vi "New Card Setup 2.vi"(0 "Yokogawa WT500 in":refnum<class "Yokogawa WT500.lvclass">, 5 "Card Array":bool[](array[boolean]), 11 "error in (no error)":errorcluster) -> (4 "Yokogawa WT500 out":refnum<class "Yokogawa WT500.lvclass">, 6 "decimal integer string":string[](array[string]), 8 "Continuous?":bool, 10 "Card chosen":i32, 14 "Time Cluster":T1, 15 "error out":errorcluster)   [LabVIEW 2012, in "Universal Power Meter.lvlib" / "Yokogawa WT500.lvlib" / "Yokogawa WT500.lvclass"]
uses:
  Yokogawa WT500.lvclass
  Universal Power Meter class/Universal Power Meter.lvclass
panel:
  in  "Current Sensor Ratio(mV/A) (10.0000)":dbl=10.0 min=0.0001 max=99999.9999 step=0.0001 format="%.4f"
  in  "Voltage Range (8: 1000V)":u16(ring)=8 items=["AUTO", "15", "30", "60", "100", "150", "300", "600", "1000", "7.5", "15", "30", "50", "75", "150", "300", "500"]
  in  "Current Range (7: 40A)":u16(ring)=7 items=["AUTO", "500 mA", "1 A", "2 A", "5 A", "10 A", "20 A", "40 A", "S-AUTO", "50 mV", "100 mV", "200 mV", "500 mV", "1 V", "2 V", "5 V", "10 V", "250 mA", "500 mA", "1 A", "2.5 A", "5 A", "10 A", "20 A", "25 mV", "50 mV", "100 mV", "250 mV", "500 mV", "1 V", "2.5 V", "5 V"]
  in  "Play Button":bool
  in  "Card to Start":u16(ring) items=["1", "2", "3"]
  in  "Measurement":enum32{"Continuous", "Timed"}(radio)
  in  "Measurement Time":dbl format="%<%H:%M:%S>t"
  in  "Warm Up Time":dbl format="%<%H:%M:%S>t"
  out "A Range (9: 5A) 2":u16(ring)=9 items=["AUTO", "10 mA", "20 mA", "50 mA", "100 mA", "200 mA", "500 mA", "1 A", "2 A", "5 A", "10 A", "20 A", "50 A", "S-AUTO", "50 mV", "100 mV", "250 mV", "500 mV", "1 V", "2.5 V", "5 V", "10 V"]
  out "V Range (12: 1000) 2":u16(ring)=9 items=["AUTO", "1.5", "3", "6", "10", "15", "30", "60", "100", "150", "300", "600", "1000"]
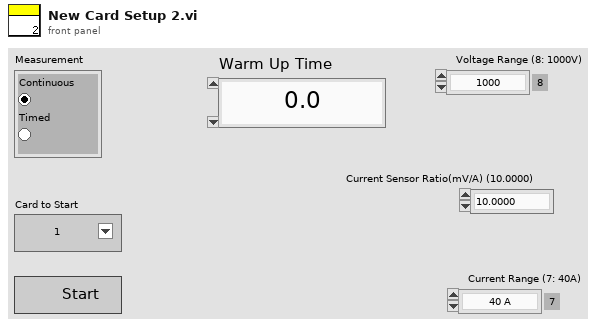
[diagram p1: front panel]
types:
  T1 = cluster{"Warm Up Time":dbl, "Measurement Time":dbl}
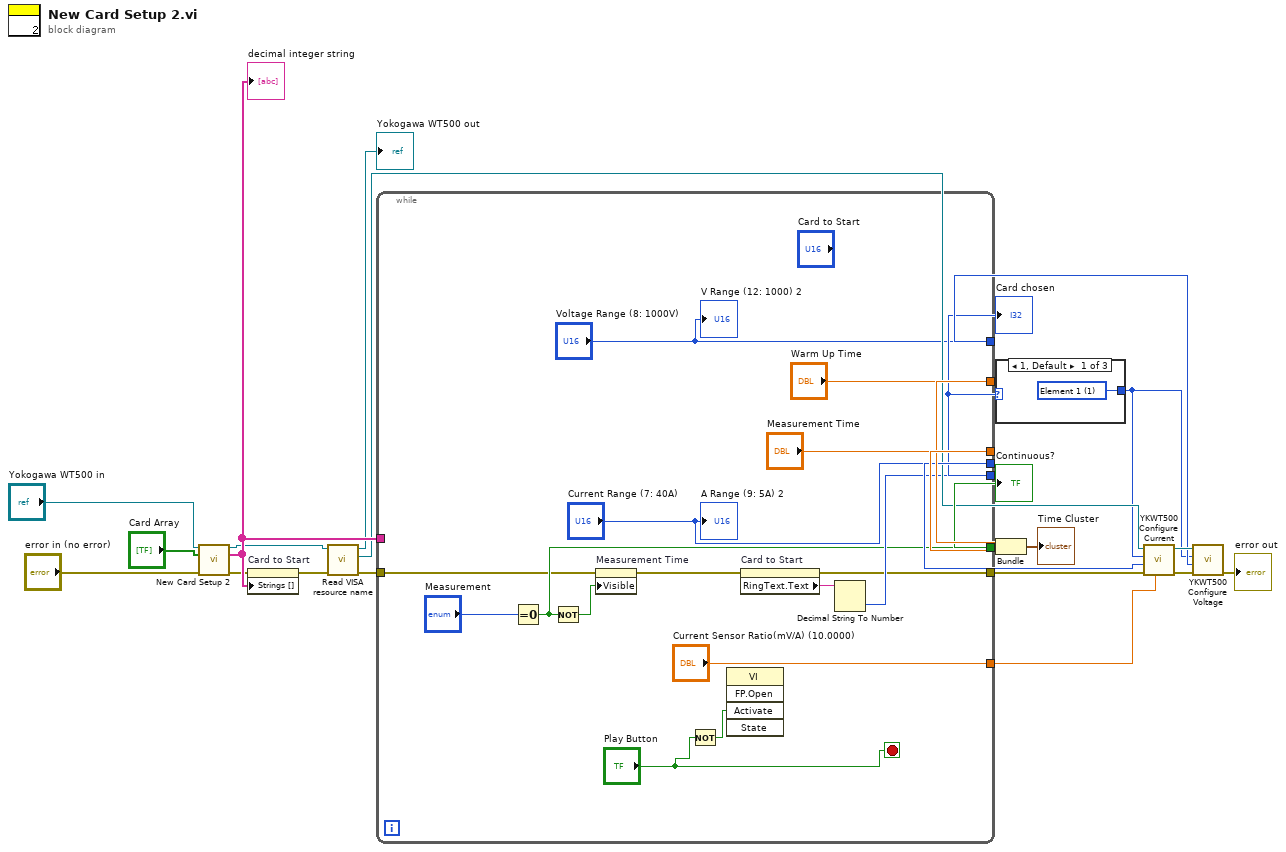
[diagram p0: block diagram]
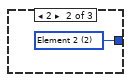
[diagram p2: hidden frame]
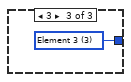
[diagram p3: hidden frame]
diagram:
  n1 = call-parent "New Card Setup 2.vi"("Generic Instrument in"="Yokogawa WT500 in", "Card Array"="Card Array", "error in (no error)"="error in (no error)") -> ("Generic Instrument out"=w9:refnum<class "Yokogawa WT500.lvclass">, "decimal integer string"=w18:string[], "error out"=w17:errorcluster)  [unwired: 7 in, 3 out]
  "decimal integer string" <- w18
  n2 = property on="Card to Start" class="Ring (strict)"(error in=w17, "Strings []"=w18) -> (error out=w7:errorcluster)  [unwired: 1 in, 1 out]
  n3 = call-dynamic "Read VISA resource name.vi"("error in (no error)"=w7, "Generic Instrument in"=w9) -> ("error out"=w6:errorcluster, "VISA resource name"=w5:refnum<visa-resource-name>, "Generic Instrument out"=→"Yokogawa WT500 out":refnum<class "Yokogawa WT500.lvclass">)  [unwired: 7 in]
  n4 = while {
    tunnel: [w37] -> w4
    tunnel: ["Measurement Time"] -> w20
    tunnel: ["Warm Up Time"] -> w19
    tunnel: [w33] -> w15
    tunnel: w18 -> [_]
    tunnel: w6 -> [w31]
    tunnel: [w29] -> w1
    tunnel: ["Current Range (7: 40A)"] -> w12
    tunnel: ["Voltage Range (8: 1000V)"] -> w11
    tunnel: ["Current Sensor Ratio(mV/A) (10.0000)"] -> w10
    stop <- "Play Button" stop-if-true
    n5 = Equal To 0?(x="Measurement") -> (x = 0?=w33:bool)
    n6 = Not(x=w33) -> (.not. x?=w32:bool)
    n7 = property on="Measurement Time" class="DigNum (strict)"(error in=w31, "Visible"=w32) -> (error out=w30:errorcluster)  [unwired: 1 in, 1 out]
    n8 = Not(x="Play Button") -> (.not. x?=w24:bool)
    n9 = invoke class="VI" method="FP.Open"("Activate"=w24) -> ()  [unwired: 4 in, 5 out]
    n10 = property on="Card to Start" class="Ring (strict)"(error in=w30) -> (error out=w29:errorcluster, "RingText.Text"=w38:string)  [unwired: 1 in, 1 out]
    n11 = Decimal String To Number(string=w38) -> (number=w37:i32)  [unwired: 2 in, 1 out]
    "A Range (9: 5A) 2" <- "Current Range (7: 40A)"
    "V Range (12: 1000) 2" <- "Voltage Range (8: 1000V)"
  }
  "Card chosen" <- w4
  "Continuous?" <- w15
  n12 = case shown="1, Default" w4 {
    tunnel: [w39 w40 w41] -> w3
    frame 1, Default {
      w39 = u16 1 items=["All", "Element 1", "Element 2", "Element 3", "Sigma"] ("Element (0: All)")
    }
    frame 2 {
      w40 = u16 2 items=["All", "Element 1", "Element 2", "Element 3", "Sigma"] ("Element (0: All)")
    }
    frame 3 {
      w41 = u16 3 items=["All", "Element 1", "Element 2", "Element 3", "Sigma"] ("Element (0: All)")
    }
  }
  n13 = Bundle("Warm Up Time"=w19, "Measurement Time"=w20) -> (→"Time Cluster":T1)  [unwired: 1 in]
  n14 = call <instrlib>:"YKWT500 Configure Current.vi"("Current Sensor Ratio(mV/A) (10.0000)"=w10, "error in (no error)"=w1, "Current Range (7: 40A)"=w12, "Element (0: All)"=w3, "VISA resource name"=w5) -> ("error out"=w13:errorcluster, "VISA resource name out"=w14:refnum<visa-resource-name>)  [unwired: 5 in]
  n15 = call <instrlib>:"YKWT500 Configure Voltage.vi"("error in (no error)"=w13, "Voltage Range (8: 1000V)"=w11, "Element (0: All)"=w3, "VISA resource name"=w14) -> ("error out"=→"error out":errorcluster)  [unwired: 6 in, 1 out]
